vi "writeToXML.vi"(8 "error in (no error)":errorcluster, 10 "ClassLabel":string, 11 "ClearPOrigin in":refnum<class "ClearPOrigin.lvclass">) -> (0 "error out":errorcluster, 2 "XML out":string, 3 "ClearPOrigin out":refnum<class "ClearPOrigin.lvclass">)   [LabVIEW 2014, in "TCSDataDefinitions.lvlib" / "TCSCommand.lvlib" / "POriginCommands.lvlib" / "ClearPOrigin.lvclass"]
uses:
  ClearPOrigin.lvclass
  ClearPOrigin.lvclass/ClearPOrigin.ctl
  POriginCommands/POriginCommands.lvclass
  <userlib>/Common/XML/XMLGenerator/XMLGenerator.lvclass
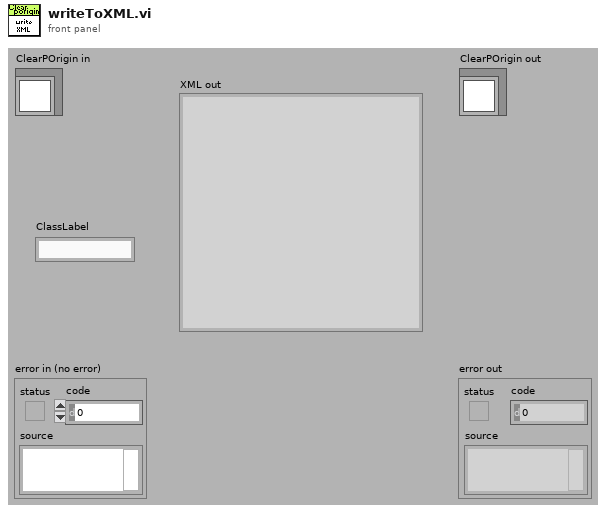
[diagram p1: front panel]
types:
  T1 = typedef "TCSDataDefinitions.lvlib/TCSCommand.lvlib/OffsetCommands.lvlib/Num2Types.ctl" = enum16{"User", "Handset", "Both"}
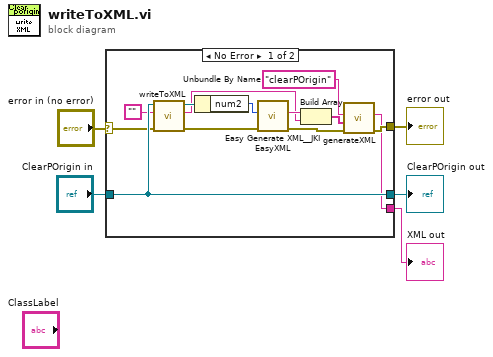
[diagram p0: block diagram]
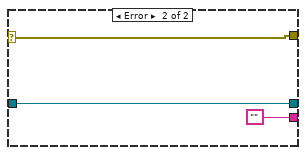
[diagram p2: hidden frame]
diagram:
  n1 = case shown="No Error" "error in (no error)" {
    selector: "error in (no error)" -> [w9 w21]
    tunnel: [w8 w21] -> w4
    tunnel: [w17 w20] -> w2
    tunnel: "ClearPOrigin in" -> [w17 w20]
    tunnel: [w7 ""] -> w1
    frame No Error {
      n2 = call-parent "writeToXML.vi"("error in (no error)"=w9, "ClassLabel"="", "POriginCommands in"=w17) -> ("error out"=w11:errorcluster, "XML out"=w12:string, "POriginCommands out"=w16:refnum<class "ClearPOrigin.lvclass">)  [unwired: 6 in]
      n3 = Unbundle By Name(w16) -> ("num2"=w18:T1)
      n4 = call <vilib>:"Easy Generate XML__JKI EasyXML.vi"("error in (no error)"=w11, "LabVIEW Data"=w18) -> ("error out"=w10:errorcluster, "XML String"=w13:string)  [unwired: 8 in]
      n5 = Build Array(w13, w12) -> (w14:string[])
      n6 = call <userlib>:"generateXML.vi"("error in"=w10, "childrenXML"=w14, "elementName"="clearPOrigin" ("Class Label")) -> ("error out"=w8:errorcluster, "XML out"=w7:string)  [unwired: 6 in, 1 out]
    }
    frame Error {
    }
  }
  "error out" <- w4
  "ClearPOrigin out" <- w2
  "XML out" <- w1
